vi "Enable GenNet Server.vi"(7 "GenNet-Server ID in":i32, 8 "error in (no error)":errorcluster, 9 "Port Number":u16, 11 "DQMH-GenNet MsgQ in":refnum<class "DQMH-GenNet Message Queue.lvclass">) -> (0 "error out":errorcluster, 5 "GenNet-Server ID out":i32)   [LabVIEW 2020, in "TCP Sever.lvlib"]
uses:
  TCP Sever.lvlib
  Libraries/hse-libraries/hse-gennet/DQMH-GenNet Message Queue.lvclass
  Libraries/hse-libraries/hse-gennet/GenNet-Server/GenNet-Server.lvlib
  Libraries/hse-libraries/hse-dqmh/Dynamic Requesters/Singleton/Status Updated Argument--cluster.ctl
  Libraries/hse-libraries/hse-dqmh/hse-dqmh-dynamicrequesters.lvlib
  Libraries/hse-libraries/hse-dqmh/Dynamic Requesters/Singleton/Error Reported Argument--cluster.ctl
  Libraries/hse-libraries/hse-dqmh/Dynamic Requesters/Singleton/Get Module Execution Status Argument--cluster.ctl
  Libraries/hse-libraries/hse-dqmh/Dynamic Requesters/Singleton/Stop Argument--cluster.ctl
  Libraries/hse-libraries/hse-dqmh/Controls/System Message Source.ctl
  Libraries/hse-libraries/hse-dqmh/hse-dqmh.lvlib
  Libraries/hse-libraries/hse-dqmh/Controls/System Message Argument--cluster.ctl
  Libraries/hse-libraries/hse-gennet/UDP Broadcasting/Generic Broadcasts.ctl
  Libraries/hse-libraries/hse-gennet/hse-gennet.lvlib
  Libraries/hse-libraries/hse-gennet/GenNet-Server/Clone Registration/Clone Registration.lvlib
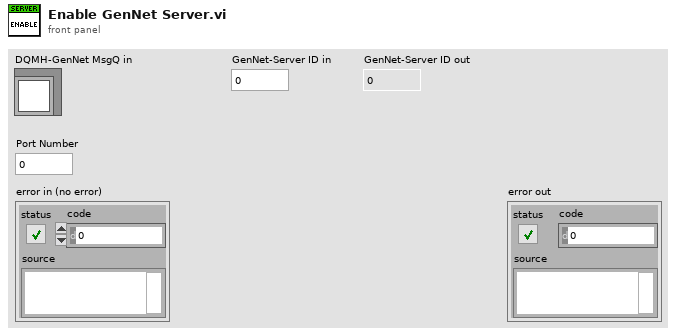
[diagram p1: front panel]
types:
  T1 = typedef "hse-gennet.lvlib/Generic Broadcasts.ctl" = cluster{"Status Updated":refnum<user-event>, "Error Reported":refnum<user-event>, "Update Module Execution Status":refnum<user-event>, "Module Did Stop":refnum<user-event>, "System Message":refnum<user-event>}
  T2 = typedef "TCP Sever.lvlib/Broadcast Events--cluster.ctl" = cluster{"Module Did Init":refnum<user-event>, "Status Updated":refnum<user-event>, "Error Reported":refnum<user-event>, "Did Something":refnum<user-event>, "Module Did Stop":refnum<user-event>, "Update Module Execution Status":refnum<user-event>, "System Messages":refnum<user-event>}
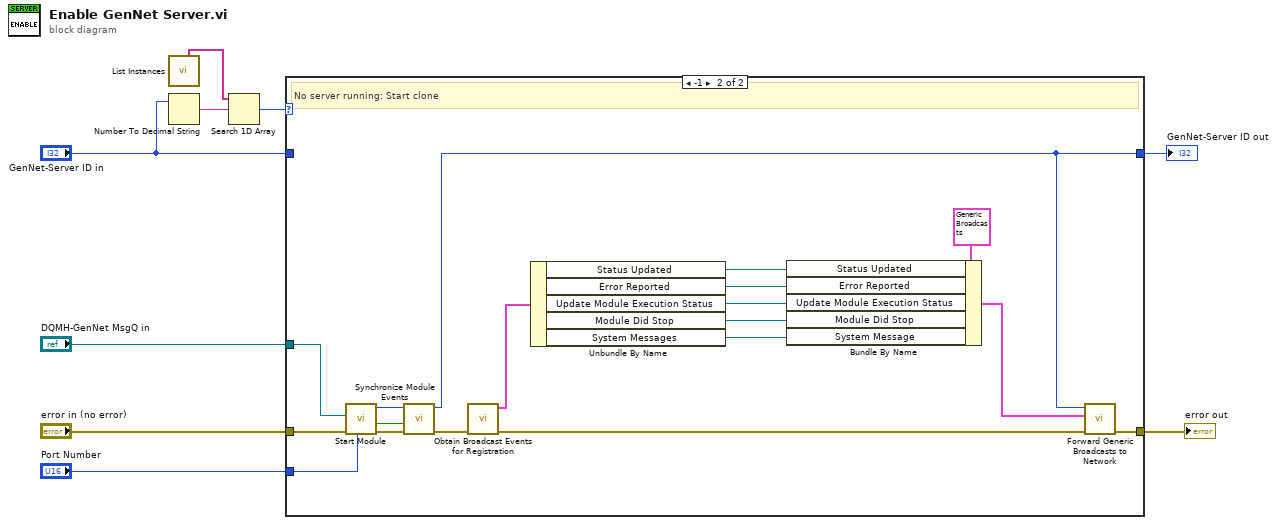
[diagram p0: block diagram]
diagram:
  n1 = call "List Instances.vi"() -> ("Instances Names"=w2:string[])  [unwired: 7 in, 4 out]
  n2 = Number To Decimal String(number="GenNet-Server ID in") -> (decimal integer string=w4:string)  [unwired: 1 in]
  n3 = Search 1D Array(1D array=w2, element=w4) -> (index of element=w1:i32)  [unwired: 1 in]
  n4 = case shown="-1" w1 {
    tunnel: "error in (no error)" -> [w11 w29]
    tunnel: "Port Number" -> [_ w28]
    tunnel: "DQMH-GenNet MsgQ in" -> [_ w23]
    tunnel: [w11 w14] -> w6
    tunnel: [w10 w12] -> w5
    tunnel: "GenNet-Server ID in" -> [w10 _]
    frame 0, Default {
      # "GenNet-Server already running..."
    }
    frame -1 {
      # "No server running: Start clone"
      n5 = call "Start Module.vi"("Port Number"=w28, "error in (no error)"=w29, "Caller MsgQ"=w23) -> ("error out"=w27:errorcluster, "Wait for Event Sync?"=w25:bool, "Module ID"=w26:i32)  [unwired: 5 in, 1 out]
      n6 = call "Synchronize Module Events.vi"("error in (no error)"=w27, "Wait for Event Sync?"=w25, "Module ID"=w26) -> ("error out"=w24:errorcluster, "Module ID (dup)"=w12:i32)  [unwired: 7 in]
      n7 = call "Obtain Broadcast Events for Registration.vi"("error in (no error)"=w24) -> ("error out"=w15:errorcluster, "TCP Sever Broadcast Events"=w22:T2)  [unwired: 8 in, 1 out]
      n8 = Unbundle By Name(w22) -> ("Status Updated"=w20:refnum<user-event>, "Error Reported"=w19:refnum<user-event>, "Update Module Execution Status"=w18:refnum<user-event>, "Module Did Stop"=w17:refnum<user-event>, "System Messages"=w16:refnum<user-event>)
      n9 = Bundle By Name(cluster=T1 {"Status Updated"=refnum, "Error Reported"=refnum, "Update Module Execution Status"=refnum, "Module Did Stop"=refnum, "System Message"=refnum} ("Generic Broadcasts"), "Status Updated"=w20, "Error Reported"=w19, "Update Module Execution Status"=w18, "Module Did Stop"=w17, "System Message"=w16) -> (w13:T1)
      n10 = call "Forward Generic Broadcasts to Network.vi"("error in (no error)"=w15, "Generic Broadcast Events"=w13, "Module ID"=w12) -> ("error out"=w14:errorcluster)  [unwired: 8 in]
    }
  }
  "GenNet-Server ID out" <- w5
  "error out" <- w6
